vi "HMI.vi"() -> ()   [LabVIEW 2019]
uses:
  Hardware/PfeifferTC110Cmds.ctl
  Hardware/PfeifferMVP15Cmds.ctl
  <vilib>/Utility/miscctls.llb/LVPointTypeDef.ctl
  <vilib>/NI/AMC/Read Termination Message.vi
  <vilib>/NI/AMC/Create Single Message.vi
  <vilib>/NI/AMC/Update Message Routing Info.vi
  <vilib>/NI/AMC/Send Message.vi
  <vilib>/NI/AMC/Globals.vi
  <vilib>/NI/AMC/AMC.lvlib
  <instrlib>/Pfeiffer Vacuum/Pfeiffer Vacuum.lvlib
panel:
  out "status":string
  in  "stop":bool
  in  "Tab Control":enum32{"RGAs", "Gas Flow", "Alarms", "Page 3"}(tab)
  in  "Ring":u16(ring)
  in  "Ack Errors":bool
  out "MainMVP  OpHrs":i32 caption="Op Hrs"
  out "MainMVP  Set Pnt RPM":i32 caption="Set Pnt RPM"
  out "Main Firm MVP":string caption="Firmware"
  out "Main Model MVP":string caption="Model"
  out "Load At Nominal":bool caption="At Nominal"
  out "Main At Nominal":bool caption="At Nominal"
  out "Main Control °C 3":i32(slide) caption="Control °C" scale=0.0..60.0
  out "Main Control °C 2":i32(slide) caption="Control °C" scale=0.0..60.0
  out "Load TMP °C":i32(slide) caption="TMP °C" scale=0.0..60.0
  out "Main TMP °C":i32(slide) caption="TMP °C" scale=0.0..60.0
  out "Load Set Pnt RPM":i32 caption="Set Pnt RPM"
  out "Main Set Pnt RPM":i32 caption="Set Pnt RPM"
  out "Load Cycles":i32 caption="Cycles"
  out "Main Cycles":i32 caption="Cycles"
  out "Load Model":string caption="Model"
  out "Main Model":string caption="Model"
  out "LoadErrorCode 2":string caption="Current Error Code"
  out "MainErrorCode":string caption="Current Error Code"
  out "Load Watts":dbl(knob) caption="Watts" scale=0.0..100.0
  out "Main Watts":dbl(knob) caption="Watts" scale=0.0..100.0
  out "Load RPM":dbl(knob) caption="RPM" scale=0.0..100000.0
  out "Main RPM":dbl(knob) caption="RPM" scale=0.0..100000.0
  in  "Load TMP Standby":bool caption="TMP Standby"
  in  "Main TMP Standby":bool caption="TMP Standby"
  in  "Load TMP Run":bool caption="TMP Run"
  in  "Main TMP Run":bool caption="TMP Run"
  out "MVP RPM":i32(knob) caption="RPM" scale=0.0..2500.0
  out "MVP Watts":i32(knob) caption="Watts" scale=0.0..100.0
  out "Load TMP °C 2":i32(slide) caption="Pmp °C" scale=0.0..60.0
  out "MVPErrorCode":string caption="Current Error Code"
  in  "Main MVP Run":bool caption="MVP Run"
  in  "MainMVP Standby":bool caption="MVP Standby"
  out "P LL":dbl format="%#_2e"
  out "Boolean 6":bool
  out "Boolean 5":bool
  out "Boolean 2":bool
  out "Watts 5":i16 caption="Volts"
  out "RF Fwd":i16
  out "RF Rlfctd":i16
  out "RF Vdc":i16
  out "Watts 4":i16 caption="Watts"
  out "Boolean 32":bool
  out "Boolean 31":bool
  out "Boolean 30":bool
  out "Boolean 29":bool
  out "Boolean 15":bool
  out "Boolean 14":bool
  out "Boolean 13":bool
  out "Boolean 12":bool
  out "Boolean 11":bool
  out "Boolean 10":bool
  out "Boolean 8":bool
  out "Watts":dbl
  out "Watts":dbl
  out "Watts":dbl
  in  "GV4":bool
  in  "GV3":bool
  in  "GV2":bool
  in  "GV1":bool
  out "Boolean":bool
  out "Unload Ch Pressure in Torr":dbl format="%.2e"
  out "MFV1 Chamber Access":bool
  out "Boolean 9":bool
  out "Boolean 7":bool
  out "Ar to MFV1":bool
  out "O2 to MFV1":bool
  out "Boolean 3":bool
  out "MFC2 Gas Spply":bool
  out "IG MFCs to GD":bool
  out "MFC3 Gas Spply":bool
  in  "GD On":bool
  in  "Blank Button 2":bool
  out "IG Chamber Access":bool
  out "MFC1":i16
  out "MFC2":sgl format="%.1f"
  out "MFC3":sgl format="%.1f"
  out "MFC3 Total":sgl format="%.1f"
  out "MFC2 Total":sgl format="%.1f"
  out "Boolean 4":bool
  in  "Blank Button 3":bool
  out "To RGA":bool
  out "Boolean 16":bool
  out "Ar Supply Target 1":bool
  out "MFC4":sgl format="%.1f"
  out "Boolean 17":bool
  out "Targ 1 Total":sgl format="%.1f"
  in  "Blank Button 4":bool
  out "Ar Supply Target 2":bool
  out "MFC5":sgl format="%.1f"
  out "Boolean 18":bool
  out "Targ 2 Total":sgl format="%.1f"
  in  "Blank Button 5":bool
  out "Ar Supply Target 3":bool
  out "MFC6":sgl format="%.1f"
  out "Boolean 19":bool
  out "Targ 3 Total":sgl format="%.1f"
  out "To RGA Main":bool caption="To RGA"
  out "N2 Vent":bool
  out "Atm Vent":bool
  out "Boolean 20":bool
  out "Boolean 21":bool
  out "Boolean 22":bool
  out "Turbo MV1":bool
  in  "LD MV1":bool
  out "Throttle Pos":dbl(knob) scale=0.0..100.0
  out "N2 Vent 2":bool caption="N2 Vent"
  out "Atm Vent 2":bool caption="Atm Vent"
  out "Boolean 23":bool
  out "Boolean 24":bool
  out "Boolean 25":bool
  out "N2 Vent 3":bool caption="N2 Vent"
  out "Atm Vent 3":bool caption="Atm Vent"
  out "Boolean 26":bool
  out "Boolean 27":bool
  out "Boolean 28":bool
  out "PLC":bool
  out "RV1":bool
  out "RV1 2":bool caption="RV3"
  out "P Mn":dbl format="%.2e"
  out "UL_vent_TO":bool
  out "UL_Rough_TO":bool
  out "RV3_Incorr_Op/CL":bool
  out "RV1_Incorr_Op/CL":bool
  out "RF_disch_MV1_Cl":bool
  out "MV1_Incorr_Op/CL":bool
  out "LL_vent_TO":bool
  out "LL_Rough_TO":bool
  out "LL_pumpdn_TO":bool
  out "FV2_Incorr_Op/CL":bool
  out "FV1_Incorr_Op/CL":bool
  out "Chmbr_vent_TO":bool
  out "Chmbr_Rough_TO":bool
  out "TMP2":bool
  out "TMP1":bool
  out "DP2":bool
  out "DP1":bool
  out "DC2B L/H Lim":bool
  out "DC2A L/H Lim":bool
  out "DC1B L/H Lim":bool
  out "DC1A L/H Lim":bool
  out "RF VDC":bool
  out "RF REV Lim":bool
  out "RF FWD Lim":bool
  out "DP3":bool
  out "RF":bool
  # "Main Chamber RGA"
  # "Load Lock RGA"
  # "Main RGA MVP"
  # "Std L"
  # "Std L"
  # "Std L"
  # "Open"
  # "Closed"
  # "SCCM"
  # "SCCM"
  # "SCCM"
  # "SCCM"
  # "Main Ch Pressure \n in Torr"
  # "Std L"
  # "SCCM"
  # "Std L"
  # "SCCM"
  # "Vacuum Alarms"
  # "Sput/Gauge Alarms"
  # "Transport Alarms"
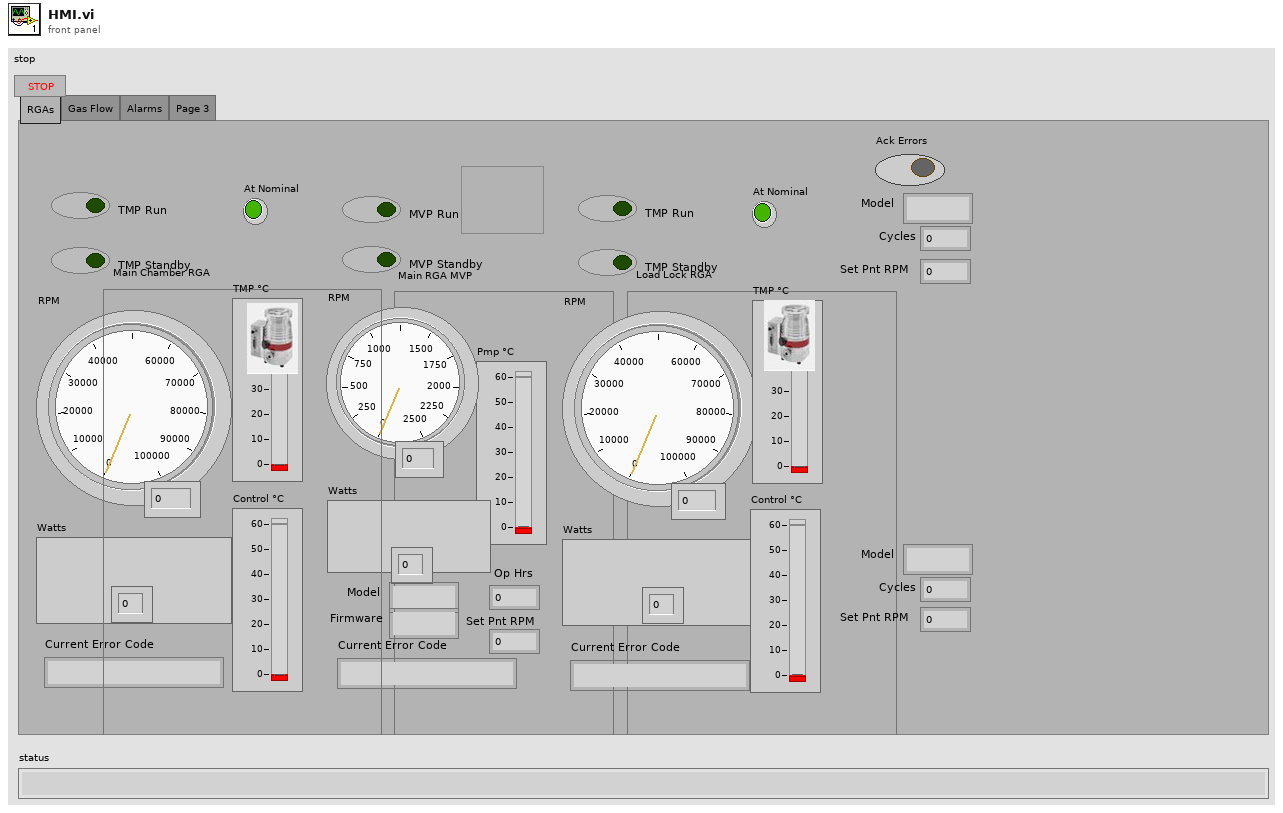
[diagram p1: front panel]
types:
  T1 = typedef "AMC.lvlib/Message Queue.ctl" = refnum<queue>
  T2 = typedef "PfeifferTC110Cmds.ctl" = enum16{"Standby", "AckError", "Run", "Motor", "SpdSwPtAtt", "ErrorCode", "OvTempElec", "OvTempPump", "SetSpdAtt", "PumpAccel", "ActualSpdHz", "DrvCurrent", "OpHrsPump", "FwVersion", "DrvVoltage", "OpHrsElec", "NominalSpd", "DrvPower", "PumpCycles", "TempElec", "TempPmpBot", "AccelDecel", "TempBearing", "TempMotor", "ElecName", "HWVersion", "SetRotSpdRPM", "ActualSpdRPM", "NominalSpdRPM"}
  T3 = typedef "PfeifferMVP15Cmds.ctl" = enum16{"Standby", "Run", "AckError", "ErrorCode", "ActualSpdHz", "DrvCurrent", "OpHrsPump", "FwVersion", "DrvVoltage", "NominalSpdHz", "DrvPower", "ElecName", "HWVersion", "ActualSpdRPM", "NominalSpdRPM", "TempPump"}
  T4 = typedef "LVPointTypeDef.ctl" = cluster{"Horizontal":i16, "Vertical":i16}
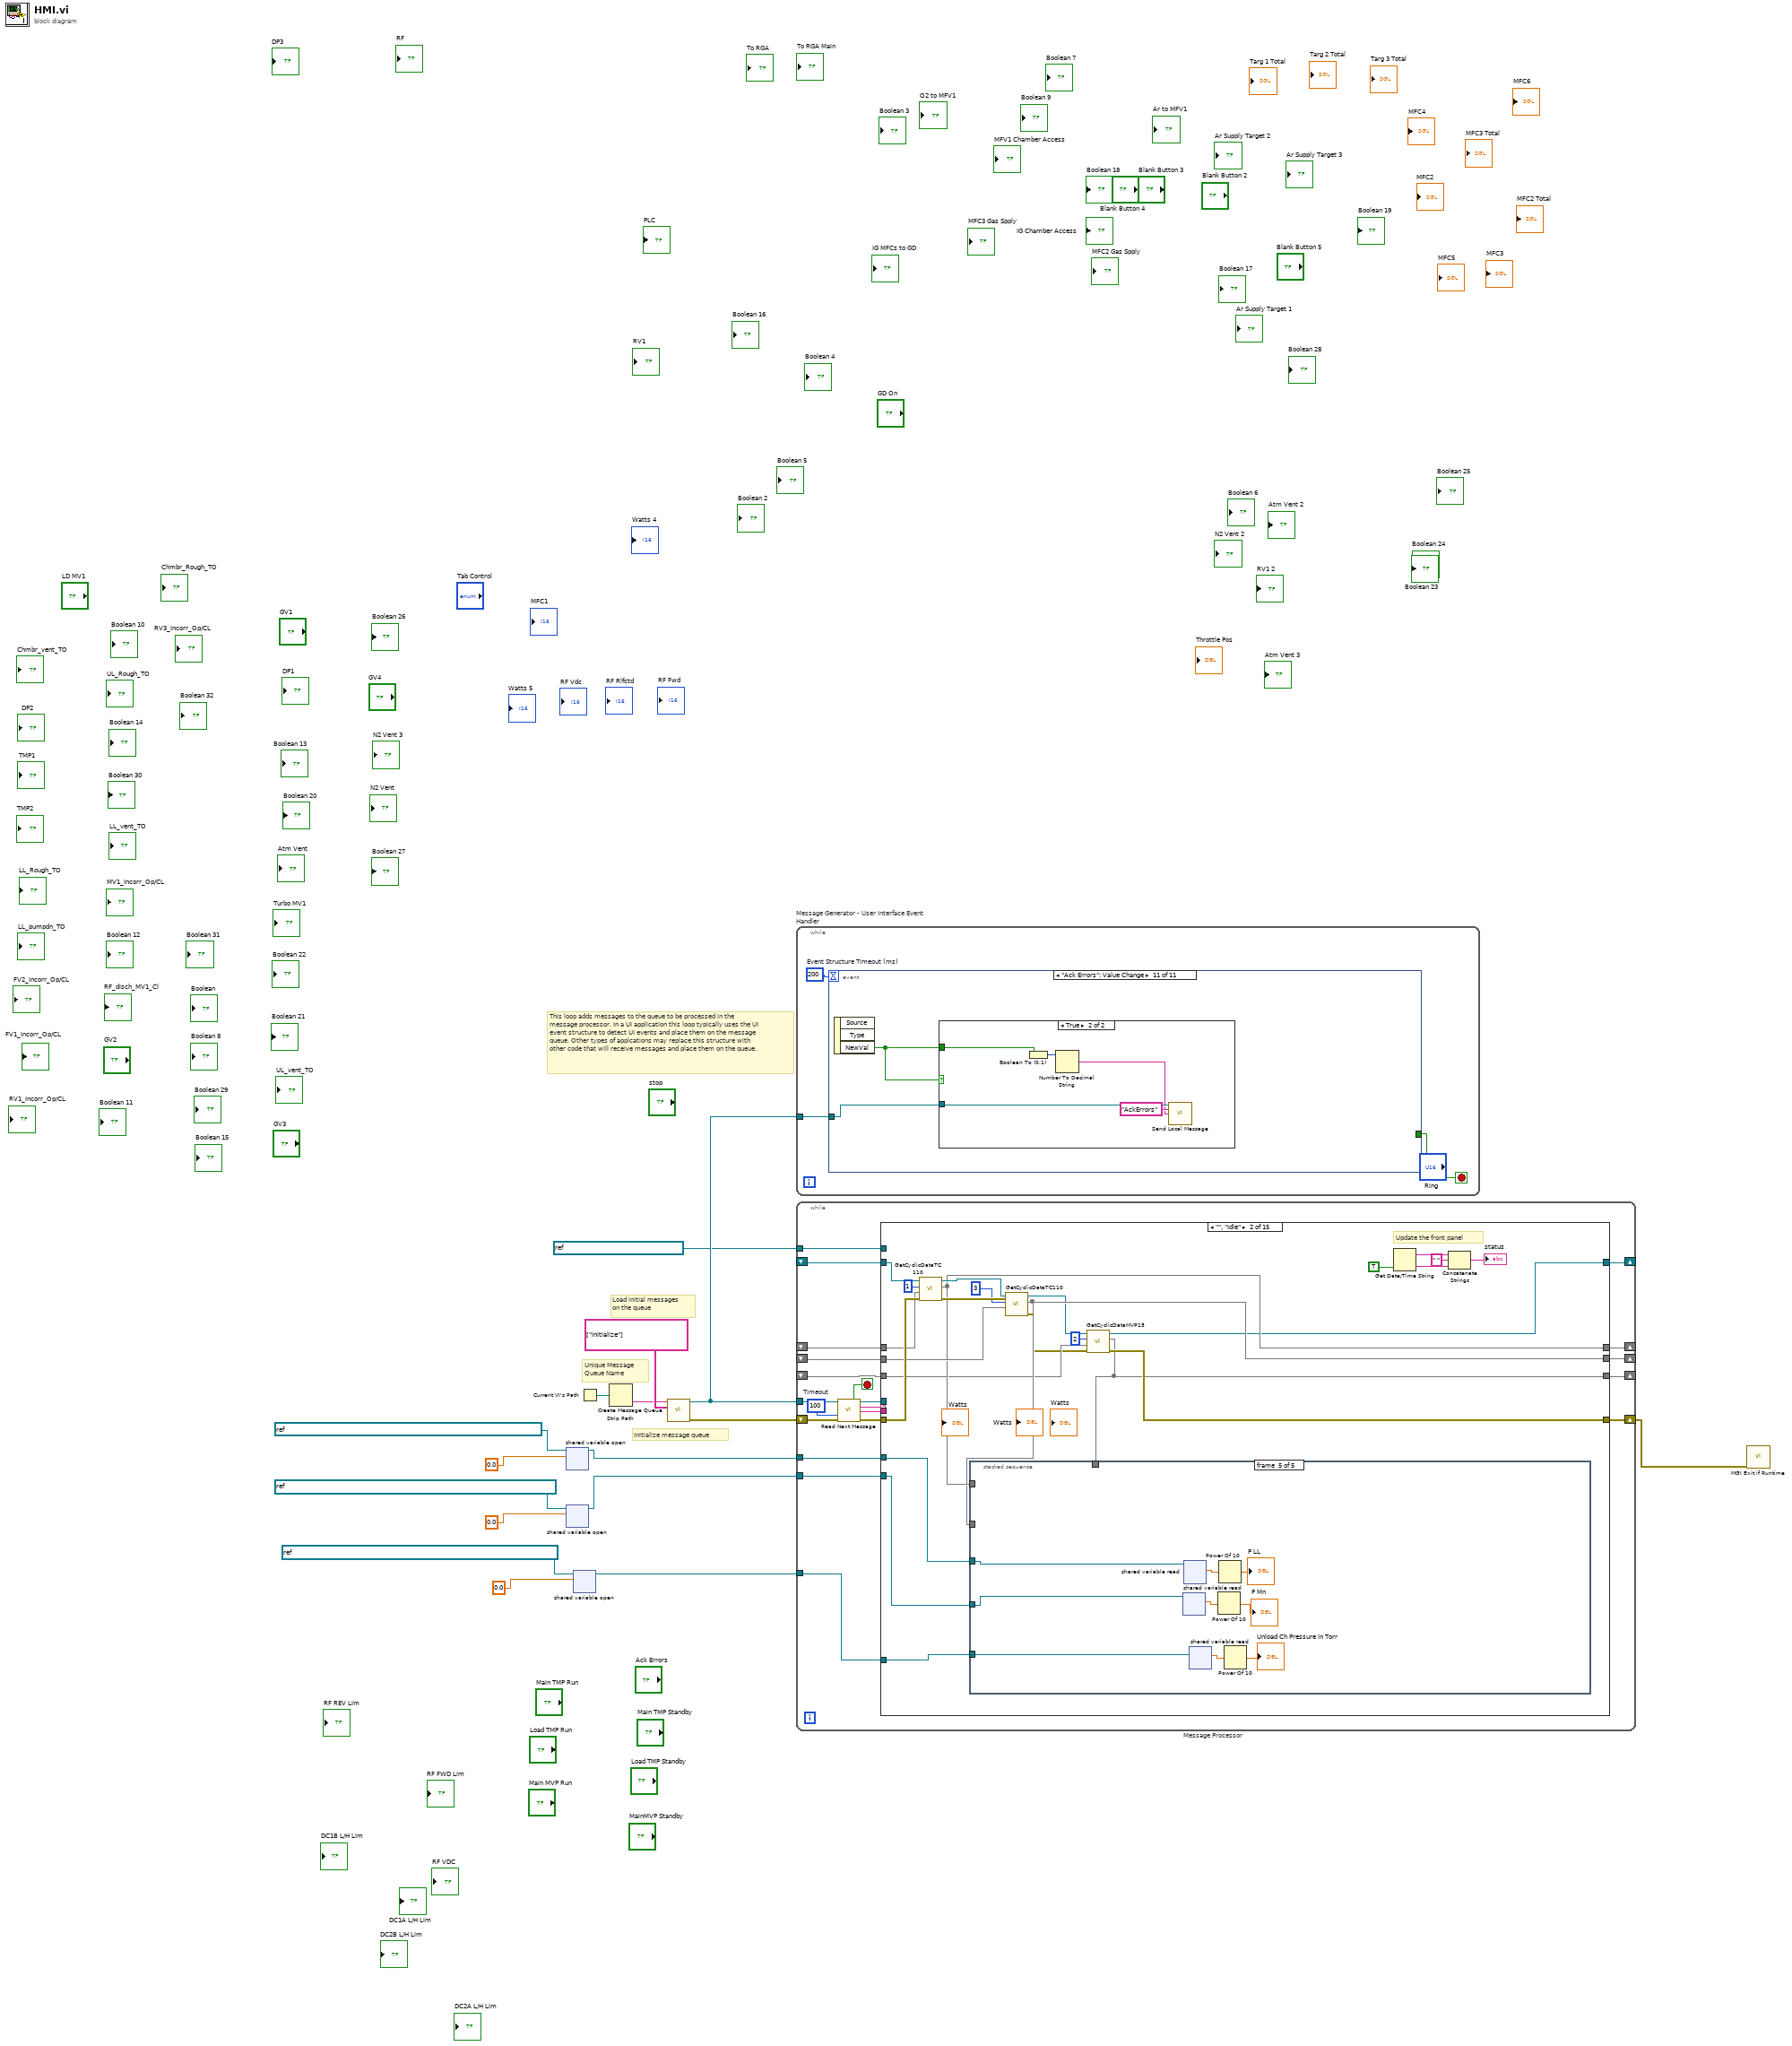
[diagram p0: block diagram]
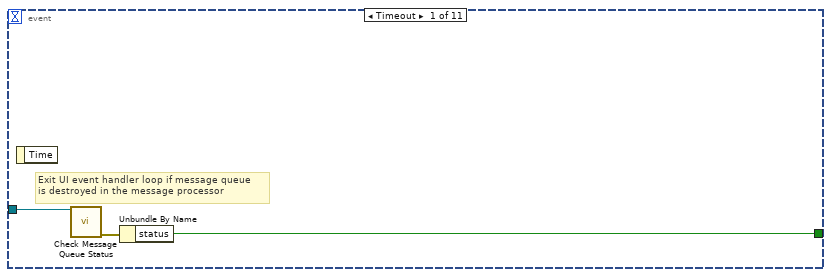
[diagram p2: hidden frame]
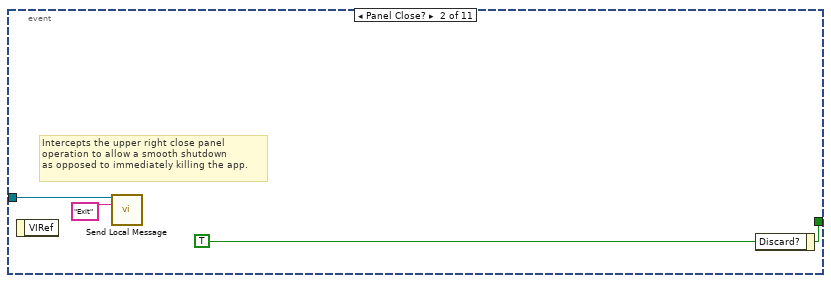
[diagram p3: hidden frame]
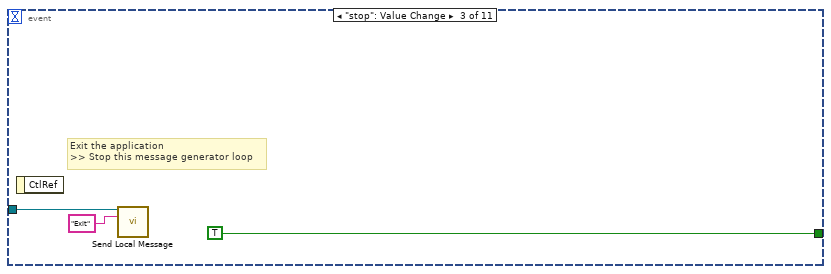
[diagram p4: hidden frame]
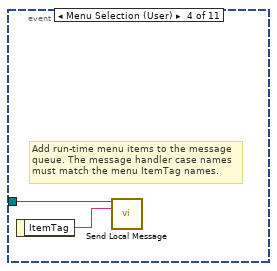
[diagram p5: hidden frame]
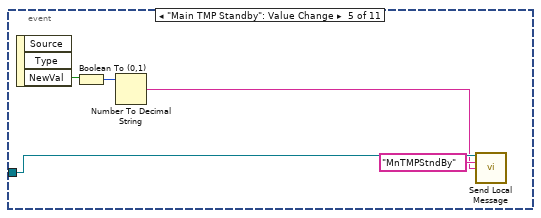
[diagram p6: hidden frame]
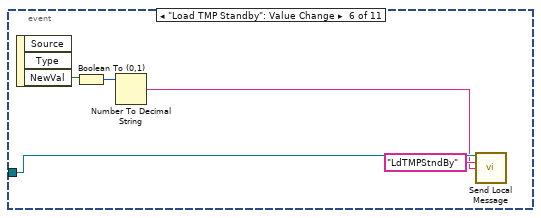
[diagram p7: hidden frame]
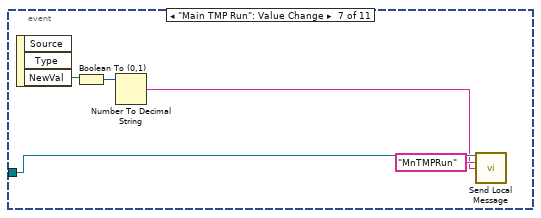
[diagram p8: hidden frame]
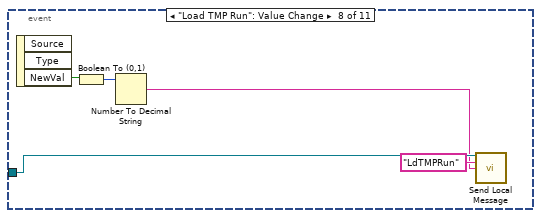
[diagram p9: hidden frame]
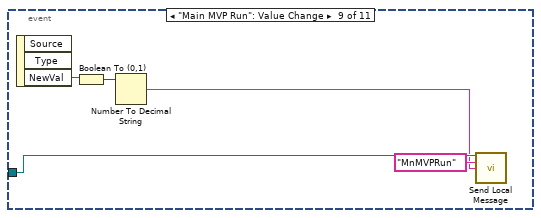
[diagram p10: hidden frame]
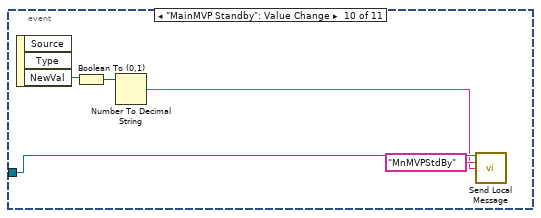
[diagram p11: hidden frame]
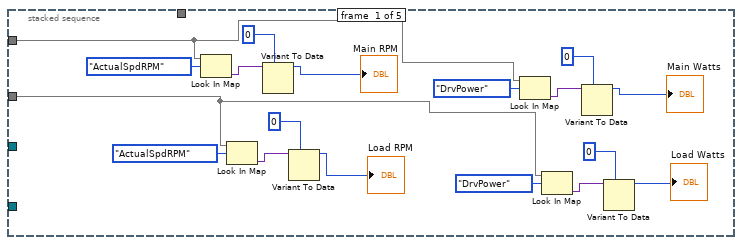
[diagram p14: hidden frame]
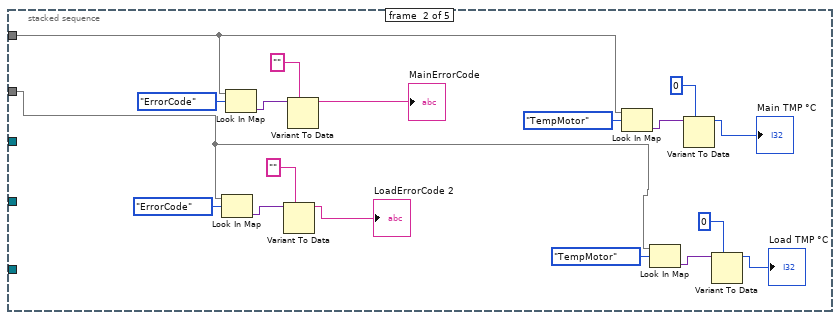
[diagram p15: hidden frame]
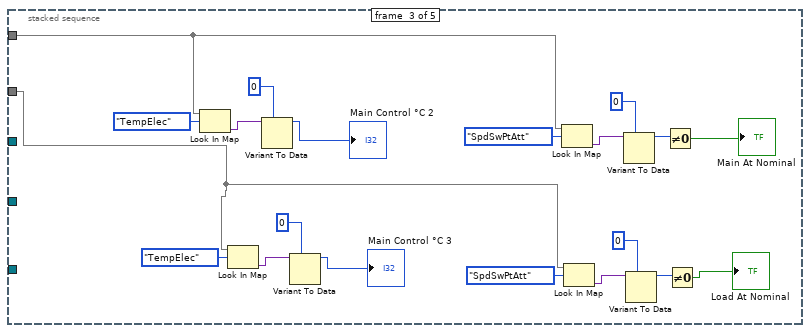
[diagram p16: hidden frame]
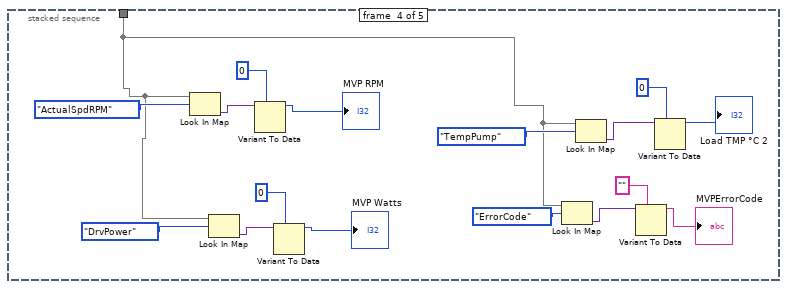
[diagram p17: hidden frame]
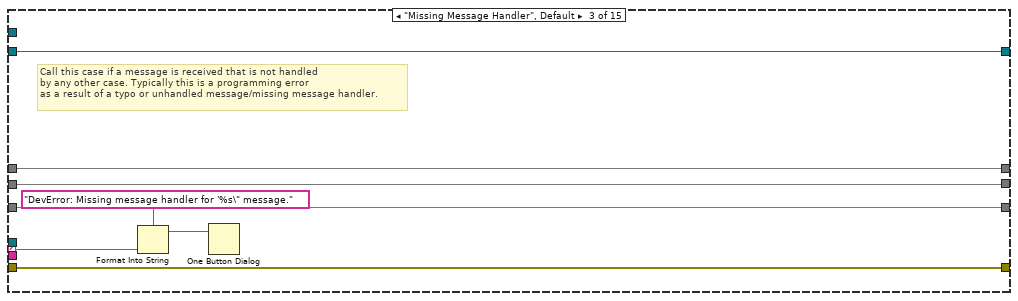
[diagram p18: hidden frame]
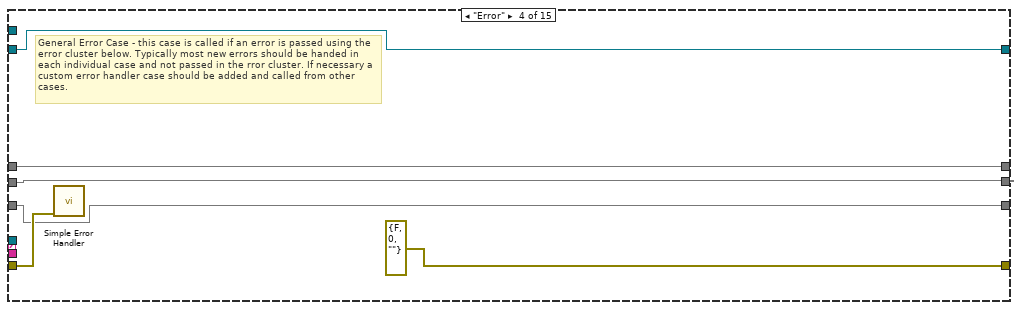
[diagram p19: hidden frame]
diagram:
  # "This loop adds messages to the queue to be processed in the message processor. In a UI application this loop typically uses the UI event structure to detect UI events and place them on the message queue. Other types of applcations may replace this structure with other code that will receive messages and place them on the queue."
  # "Initialize message queue"
  # "Unique Message\nQueue Name"
  # "Load initial messages\non the queue"
  n1 = shared-variable-open(refnum<k21> "ni.var.psp://huniopc01/CDL0097 scada tags/Load_Lock_Pressure" ("shared variable refnum in"), 0.0) -> (w5:refnum<k21>)  [unwired: 2 in, 1 out]
  n2 = shared-variable-open(refnum<k21> "ni.var.psp://huniopc01/CDL0097 scada tags/Main_Chamber_Log10P" ("shared variable refnum in"), 0.0) -> (w4:refnum<k21>)  [unwired: 2 in, 1 out]
  n3 = shared-variable-open(refnum<k21> "ni.var.psp://huniopc01/CDL0097 scada tags/Unload_Lock_Pressure" ("shared variable refnum in"), 0.0) -> (w1:refnum<k21>)  [unwired: 2 in, 1 out]
  n4 = Current VI's Path() -> (path=w12:path)
  n5 = Strip Path(path=w12) -> (name=w15:string)  [unwired: 1 out]
  n6 = call <vilib>:"Create Message Queue.vi"("message queue name"=w15, "initial message names"=string[] ["Initialize"]) -> ("message queue out"=w14:T1, "error out"=w13:errorcluster)  [unwired: 12 in]
  n7 = while "Message Generator - User Interface Event Handler" {
    tunnel: w14 -> [w17]
    stop <- w18 stop-if-true
    w19 = 200  # Event Structure Timeout (ms)
    n8 = event shown="[10] \"Ack Errors\": Value Change" {
      selector: _ -> [_ _ _ _ _ _ _ _ _ _ _]
      dyn-events: _ -> [_ _ _ _ _ _ _ _ _ _ _]
      timeout: w19 -> [_ _ _ _ _ _ _ _ _ _ _]
      tunnel: [w20 w25 TRUE ("Discard?") _ _ _ _ _ _ _ _] -> w18
      tunnel: w17 -> [w21 w23 w26 w29 w35 w40 w45 w50 w55 w60 w62]
      event Timeout {
        # "Exit UI event handler loop if message queue\nis destroyed in the message processor"
        n9 = event-data() -> ()  [unwired: 2 out]
        n10 = call <vilib>:"Check Message Queue Status.vi"("message queue in"=w21) -> ("error out"=w22:errorcluster)  [unwired: 10 in, 4 out]
        n11 = Unbundle By Name(w22) -> ("status"=w20:bool)
      }
      event Panel Close? {
        w25 = TRUE ("Discard?")
        # "Intercepts the upper right close panel\noperation to allow a smooth shutdown\nas opposed to immediately killing the app."
        n12 = event-data() -> ()  [unwired: 2 out]
        n13 = call <vilib>:"Send Local Message.vi"("message queue in"=w23, "message name"="Exit") -> ()  [unwired: 11 in, 3 out]
        n14 = event-data("Discard?"=w25) -> ()  [unwired: 1 in, 1 out]
      }
      event "stop": Value Change {
        # "Exit the application\n>> Stop this message generator loop"
        n15 = event-data() -> ()  [unwired: 2 out]
        n16 = call <vilib>:"Send Local Message.vi"("message queue in"=w26, "message name"="Exit") -> ()  [unwired: 11 in, 3 out]
      }
      event Menu Selection (User) {
        # "Add run-time menu items to the message\nqueue. The message handler case names must match the menu ItemTag names."
        n17 = event-data() -> ("ItemTag"=w30:string)  [unwired: 1 out]
        n18 = call <vilib>:"Send Local Message.vi"("message queue in"=w29, "message name"=w30) -> ()  [unwired: 11 in, 3 out]
      }
      event "Main TMP Standby": Value Change {
        n19 = event-data() -> ("NewVal"=w34:bool)  [unwired: 3 out]
        n20 = Boolean To (0,1)(Boolean=w34) -> (0, 1=w32:i16)
        n21 = Number To Decimal String(number=w32) -> (decimal integer string=w31:string)  [unwired: 1 in]
        n22 = call <vilib>:"Send Local Message.vi"("message queue in"=w35, "message name"="MnTMPStndBy", "message value"=w31) -> ()  [unwired: 10 in, 3 out]
      }
      event "Load TMP Standby": Value Change {
        n23 = event-data() -> ("NewVal"=w39:bool)  [unwired: 3 out]
        n24 = Boolean To (0,1)(Boolean=w39) -> (0, 1=w37:i16)
        n25 = Number To Decimal String(number=w37) -> (decimal integer string=w36:string)  [unwired: 1 in]
        n26 = call <vilib>:"Send Local Message.vi"("message queue in"=w40, "message name"="LdTMPStndBy", "message value"=w36) -> ()  [unwired: 10 in, 3 out]
      }
      event "Main TMP Run": Value Change {
        n27 = event-data() -> ("NewVal"=w44:bool)  [unwired: 3 out]
        n28 = Boolean To (0,1)(Boolean=w44) -> (0, 1=w42:i16)
        n29 = Number To Decimal String(number=w42) -> (decimal integer string=w41:string)  [unwired: 1 in]
        n30 = call <vilib>:"Send Local Message.vi"("message queue in"=w45, "message name"="MnTMPRun", "message value"=w41) -> ()  [unwired: 10 in, 3 out]
      }
      event "Load TMP Run": Value Change {
        n31 = event-data() -> ("NewVal"=w49:bool)  [unwired: 3 out]
        n32 = Boolean To (0,1)(Boolean=w49) -> (0, 1=w47:i16)
        n33 = Number To Decimal String(number=w47) -> (decimal integer string=w46:string)  [unwired: 1 in]
        n34 = call <vilib>:"Send Local Message.vi"("message queue in"=w50, "message name"="LdTMPRun", "message value"=w46) -> ()  [unwired: 10 in, 3 out]
      }
      event "Main MVP Run": Value Change {
        n35 = event-data() -> ("NewVal"=w54:bool)  [unwired: 3 out]
        n36 = Boolean To (0,1)(Boolean=w54) -> (0, 1=w52:i16)
        n37 = Number To Decimal String(number=w52) -> (decimal integer string=w51:string)  [unwired: 1 in]
        n38 = call <vilib>:"Send Local Message.vi"("message queue in"=w55, "message name"="MnMVPRun", "message value"=w51) -> ()  [unwired: 10 in, 3 out]
      }
      event "MainMVP Standby": Value Change {
        n39 = event-data() -> ("NewVal"=w59:bool)  [unwired: 3 out]
        n40 = Boolean To (0,1)(Boolean=w59) -> (0, 1=w57:i16)
        n41 = Number To Decimal String(number=w57) -> (decimal integer string=w56:string)  [unwired: 1 in]
        n42 = call <vilib>:"Send Local Message.vi"("message queue in"=w60, "message name"="MnMVPStdBy", "message value"=w56) -> ()  [unwired: 10 in, 3 out]
      }
      event "Ack Errors": Value Change {
        n43 = event-data() -> ("NewVal"=w61:bool)  [unwired: 3 out]
        n44 = case shown="True" w61 {
          tunnel: w62 -> [_ w67]
          tunnel: w61 -> [_ w66]
          frame False {
          }
          frame True {
            n45 = Boolean To (0,1)(Boolean=w66) -> (0, 1=w64:i16)
            n46 = Number To Decimal String(number=w64) -> (decimal integer string=w63:string)  [unwired: 1 in]
            n47 = call <vilib>:"Send Local Message.vi"("message queue in"=w67, "message name"="AckErrors", "message value"=w63) -> ()  [unwired: 10 in, 3 out]
          }
        }
      }
    }
  }
  n48 = while "Message Processor" {
    shift-left: w13 -> [w84]
    shift-right: [w88] -> w10
    tunnel: w14 -> [w85]
    tunnel: refnum<visa-resource-name> "visa://Z016807/ASRL5::INSTR" ("VISA resource name") -> [w79]
    shift-right: [w78] -> _
    shift-left: _ -> [w75]
    shift-right: [w77] -> _
    shift-left: _ -> [w73]
    shift-right: [w76] -> _
    shift-left: _ -> [w74]
    tunnel: w5 -> [w72]
    tunnel: w4 -> [w71]
    shift-right: [w70] -> _
    shift-left: _ -> [w69]
    tunnel: w1 -> [w68]
    stop <- w87 stop-if-true
    w80 = 100  # Timeout
    n49 = call <vilib>:"Read Next Message.vi"("message queue in"=w85, "timeout (1 ms)"=w80, "error in"=w84) -> ("exit process?"=w87:bool, "message queue out"=w86:T1, "message name"=w82:string, "message value"=w81:string, "error out"=w83:errorcluster)  [unwired: 5 in, 3 out]
    n50 = case shown="\"\", \"Idle\"" w82 {
      selector: w82 -> [_ _ w207 _ _ _ _ _ _ _ _ _ _ _ _]
      tunnel: w86 -> [_ _ _ _ _ _ w333 _ _ _ _ _ _ _ _]
      tunnel: w83 -> [w93 w111 w208 w213 w219 w245 w334 w340 w351 w366 w381 w396 w406 w421 w444]
      tunnel: [w93 w96 w208 errorcluster {"status"=FALSE, "code"=0, "source"=""} ("error out") w219 w222 w331 w340 w343 w358 w373 w388 w401 w416 w435] -> w88
      tunnel: w81 -> [_ _ _ _ _ _ _ _ w349 w364 w379 w394 w414 w429 _]
      tunnel: w79 -> [_ _ _ _ _ w246 _ _ _ _ _ _ _ _ _]
      tunnel: [w92 w100 w204 w210 w216 w221 w330 w337 w350 w365 w380 w395 w410 w425 w433] -> w78
      tunnel: [w90 w104 w202 w211 w218 w230 w328 w339 w355 w370 w385 w400 w415 w430 w442] -> w77
      tunnel: [w91 w105 w203 w212 w217 w231 w329 w338 w342 w357 w372 w387 w412 w427 w443] -> w76
      tunnel: w75 -> [w92 w113 w204 w210 w216 _ w330 w337 w353 w368 w383 w398 w411 w426 w446]
      tunnel: w74 -> [w91 w110 w203 w212 w217 w233 w329 w338 w346 w361 w376 w391 w412 w427 w443]
      tunnel: w73 -> [w90 w108 w202 w211 w218 w232 w328 w339 w355 w370 w385 w400 w415 w430 w442]
      tunnel: w72 -> [_ w102 _ _ _ _ _ _ _ _ _ _ _ _ _]
      tunnel: w71 -> [_ w103 _ _ _ _ _ _ _ _ _ _ _ _ _]
      tunnel: [w89 w95 w201 w209 w215 w220 w327 w336 w341 w356 w371 w386 w402 w417 w434] -> w70
      tunnel: w69 -> [w89 w99 w201 w209 w215 _ w327 w336 w341 w356 w371 w386 w404 w419 w434]
      tunnel: w68 -> [_ w94 _ _ _ _ _ _ _ _ _ _ _ _ _]
      frame "---------- Framework Operations ----------" {
        # "Dummy case to add a seperator in the Case Structure menu"
      }
      frame "", "Idle" {
        # "Update the front panel"
        n51 = call "GetCyclicDataTC110.vi"("error in (no error)"=w111, "Map"=w110, "Adress of unit"=u16 1, "VISA Refnum in"=w113) -> ("error out"=w109:errorcluster, "Map 2"=w105:map{T2, variant}, "VISA session out"=w106:refnum<visa-resource-name>)  [unwired: 5 in]
        n52 = call "GetCyclicDataTC110.vi"("error in (no error)"=w109, "Map"=w108, "Adress of unit"=u16 3, "VISA Refnum in"=w106) -> ("error out"=w97:errorcluster, "Map 2"=w104:map{T2, variant}, "VISA session out"=w101:refnum<visa-resource-name>)  [unwired: 5 in]
        n53 = call "GetCyclicDataMVP15.vi"("error In"=w97, "Map In"=w99, "Adress"=u16 2, "VISA session"=w101) -> ("error out"=w96:errorcluster, "Map"=w95:map{T3, variant}, "VISA session Out"=w100:refnum<visa-resource-name>)  [unwired: 5 in]
        n54 = stacked-sequence {
          tunnel: w105 -> [w125 w140 w164 _ _]
          tunnel: w104 -> [w120 w139 w156 _ _]
          tunnel: w103 -> [_ _ _ _ w195]
          tunnel: w102 -> [_ _ _ _ w196]
          tunnel: w95 -> [_ _ _ w178 _]
          tunnel: w94 -> [_ _ _ _ w193]
          frame #0 {
            n55 = Look In Map(map=w125, key=PfeifferTC110Cmds."ActualSpdRPM") -> (value=w134:variant)  [unwired: 1 in, 1 out]
            n56 = Look In Map(map=w120, key=PfeifferTC110Cmds."ActualSpdRPM") -> (value=w130:variant)  [unwired: 1 in, 1 out]
            n57 = Variant To Data(type=0, Variant=w134) -> (data=→"Main RPM":i32)  [unwired: 1 in, 1 out]
            n58 = Variant To Data(type=0, Variant=w130) -> (data=→"Load RPM":i32)  [unwired: 1 in, 1 out]
            n59 = Look In Map(map=w125, key=PfeifferTC110Cmds."DrvPower") -> (value=w126:variant)  [unwired: 1 in, 1 out]
            n60 = Look In Map(map=w120, key=PfeifferTC110Cmds."DrvPower") -> (value=w121:variant)  [unwired: 1 in, 1 out]
            n61 = Variant To Data(type=0, Variant=w126) -> (data=→"Main Watts":i32)  [unwired: 1 in, 1 out]
            n62 = Variant To Data(type=0, Variant=w121) -> (data=→"Load Watts":i32)  [unwired: 1 in, 1 out]
          }
          frame #1 {
            n63 = Look In Map(map=w139, key=PfeifferTC110Cmds."ErrorCode") -> (value=w149:variant)  [unwired: 1 in, 1 out]
            n64 = Look In Map(map=w140, key=PfeifferTC110Cmds."ErrorCode") -> (value=w153:variant)  [unwired: 1 in, 1 out]
            n65 = Variant To Data(type="", Variant=w149) -> (data=→"LoadErrorCode 2":string)  [unwired: 1 in, 1 out]
            n66 = Variant To Data(type="", Variant=w153) -> (data=→"MainErrorCode":string)  [unwired: 1 in, 1 out]
            n67 = Look In Map(map=w140, key=PfeifferTC110Cmds."TempMotor") -> (value=w145:variant)  [unwired: 1 in, 1 out]
            n68 = Look In Map(map=w139, key=PfeifferTC110Cmds."TempMotor") -> (value=w142:variant)  [unwired: 1 in, 1 out]
            n69 = Variant To Data(type=0, Variant=w145) -> (data=→"Main TMP °C":i32)  [unwired: 1 in, 1 out]
            n70 = Variant To Data(type=0, Variant=w142) -> (data=→"Load TMP °C":i32)  [unwired: 1 in, 1 out]
          }
          frame #2 {
            n71 = Look In Map(map=w164, key=PfeifferTC110Cmds."TempElec") -> (value=w173:variant)  [unwired: 1 in, 1 out]
            n72 = Look In Map(map=w156, key=PfeifferTC110Cmds."TempElec") -> (value=w170:variant)  [unwired: 1 in, 1 out]
            n73 = Variant To Data(type=0, Variant=w173) -> (data=→"Main Control °C 2":i32)  [unwired: 1 in, 1 out]
            n74 = Variant To Data(type=0, Variant=w170) -> (data=→"Main Control °C 3":i32)  [unwired: 1 in, 1 out]
            n75 = Look In Map(map=w164, key=PfeifferTC110Cmds."SpdSwPtAtt") -> (value=w163:variant)  [unwired: 1 in, 1 out]
            n76 = Look In Map(map=w156, key=PfeifferTC110Cmds."SpdSwPtAtt") -> (value=w158:variant)  [unwired: 1 in, 1 out]
            n77 = Variant To Data(type=0, Variant=w163) -> (data=w162:i32)  [unwired: 1 in, 1 out]
            n78 = Variant To Data(type=0, Variant=w158) -> (data=w157:i32)  [unwired: 1 in, 1 out]
            n79 = Not Equal To 0?(x=w162) -> (x != 0?=→"Main At Nominal":bool)
            n80 = Not Equal To 0?(x=w157) -> (x != 0?=→"Load At Nominal":bool)
          }
          frame #3 {
            n81 = Look In Map(map=w178, key=PfeifferMVP15Cmds."ActualSpdRPM") -> (value=w190:variant)  [unwired: 1 in, 1 out]
            n82 = Look In Map(map=w178, key=PfeifferMVP15Cmds."DrvPower") -> (value=w186:variant)  [unwired: 1 in, 1 out]
            n83 = Variant To Data(type=0, Variant=w190) -> (data=→"MVP RPM":i32)  [unwired: 1 in, 1 out]
            n84 = Variant To Data(type=0, Variant=w186) -> (data=→"MVP Watts":i32)  [unwired: 1 in, 1 out]
            n85 = Look In Map(map=w178, key=PfeifferMVP15Cmds."ErrorCode") -> (value=w177:variant)  [unwired: 1 in, 1 out]
            n86 = Look In Map(map=w178, key=PfeifferMVP15Cmds."TempPump") -> (value=w181:variant)  [unwired: 1 in, 1 out]
            n87 = Variant To Data(type="", Variant=w177) -> (data=→"MVPErrorCode":string)  [unwired: 1 in, 1 out]
            n88 = Variant To Data(type=0, Variant=w181) -> (data=→"Load TMP °C 2":i32)  [unwired: 1 in, 1 out]
          }
          frame #4 {
            n89 = shared-variable-read(w195) -> (w198:dbl)  [unwired: 1 in, 3 out]
            n90 = shared-variable-read(w196) -> (w200:dbl)  [unwired: 1 in, 3 out]
            n91 = shared-variable-read(w193) -> (w194:dbl)  [unwired: 1 in, 3 out]
            n92 = Power Of 10(x=w198) -> (10^x=→"P Mn":dbl)
            n93 = Power Of 10(x=w200) -> (10^x=→"P LL":dbl)
            n94 = Power Of 10(x=w194) -> (10^x=→"Unload Ch Pressure in Torr":dbl)
          }
        }
        n95 = Get Date/Time String(want seconds? (F)=TRUE) -> (date string=w118:string, time string=w117:string)  [unwired: 2 out]
        n96 = Concatenate Strings(w118, " " ("string"), w117) -> (→"status":string)
      }
      frame "Missing Message Handler", Default {
        # "Call this case if a message is received that is not handled \nby any other case. Typically this is a programming error\nas a result of a typo or unhandled message/missing message handler."
        n97 = Format Into String(format string="DevError: Missing message handler for '%s\" message." ("message"), w207) -> (resulting string=w205:string)  [unwired: 2 in, 1 out]
        n98 = One Button Dialog(message=w205) -> ()  [unwired: 2 out]
      }
      frame "Error" {
        # "General Error Case - this case is called if an error is passed using the error cluster below. Typically most new errors should be handed in each individual case and not passed in the rror cluster. If necessary a custom error handler case should be added and called from other cases."
        n99 = call <vilib>:"Simple Error Handler.vi"("error in (no error)"=w213) -> ()  [unwired: 1 in, 8 out]
      }
      frame "---------- Generic Operations ----------" {
        # "Dummy case to add a seperator in the Case Structure menu"
      }
      frame "Initialize" {
        w225 = u16 2 ("Adress")
        w236 = u16 3 ("Adress of unit")
        w242 = u16 1 ("Adress of unit")
        # "Initialize the state variables and user interface"
        n100 = property on="Pane" class="Pane"("Origin"=T4 {"Horizontal"=0, "Vertical"=0}) -> ()  [unwired: 2 in, 2 out]
        n101 = VISA Open(VISA resource name=w246) -> (VISA resource name=w248:refnum<visa-resource-name>, error out=w247:errorcluster)  [unwired: 4 in]
        n102 = call <instrlib>:"PV Initialize.vi"("error in (no error)"=w247, "VISA session in"=w248) -> ("VISA session out"=w241:refnum<visa-resource-name>)  [unwired: 8 in, 1 out]
        n103 = call "GetInitialDataTC110.vi"("error in (no error)"=w245, "Map"=w233, "Adress of unit"=w242, "VISA Refnum in"=w241) -> ("error out"=w244:errorcluster, "data map"=w235:map{T2, variant}, "VISA session out"=w240:refnum<visa-resource-name>)  [unwired: 5 in]
        n104 = call "GetInitialDataTC110.vi"("error in (no error)"=w244, "Map"=w232, "Adress of unit"=w236, "VISA Refnum in"=w240) -> ("error out"=w243:errorcluster, "data map"=w234:map{T2, variant}, "VISA session out"=w239:refnum<visa-resource-name>)  [unwired: 5 in]
        n105 = call "GetCyclicDataTC110.vi"("error in (no error)"=w243, "Map"=w235, "Adress of unit"=w242, "VISA Refnum in"=w239) -> ("error out"=w238:errorcluster, "Map 2"=w231:map{T2, variant}, "VISA session out"=w237:refnum<visa-resource-name>)  [unwired: 5 in]
        n106 = call "GetCyclicDataTC110.vi"("error in (no error)"=w238, "Map"=w234, "Adress of unit"=w236, "VISA Refnum in"=w237) -> ("error out"=w227:errorcluster, "Map 2"=w230:map{T2, variant}, "VISA session out"=w228:refnum<visa-resource-name>)  [unwired: 5 in]
        n107 = call "GetInitialDataMVP15.vi"("error In"=w227, "Adress"=w225, "VISA session"=w228) -> ("error out"=w223:errorcluster, "Map"=w224:map{T3, variant}, "VISA session Out"=w226:refnum<visa-resource-name>)  [unwired: 6 in]
        n108 = call "GetCyclicDataMVP15.vi"("error In"=w223, "Map In"=w224, "Adress"=w225, "VISA session"=w226) -> ("error out"=w222:errorcluster, "Map"=w220:map{T3, variant}, "VISA session Out"=w221:refnum<visa-resource-name>)  [unwired: 5 in]
        n109 = stacked-sequence {
          tunnel: w231 -> [w256 w278 w290 _ _]
          tunnel: w230 -> [w250 w272 w289 _ _]
          tunnel: w220 -> [_ _ _ w302 w317]
          frame #0 {
            n110 = Look In Map(map=w250, key=PfeifferTC110Cmds."Run") -> (value=w262:variant)  [unwired: 1 in, 1 out]
            n111 = Look In Map(map=w256, key=PfeifferTC110Cmds."Run") -> (value=w269:variant)  [unwired: 1 in, 1 out]
            n112 = Variant To Data(type=0, Variant=w269) -> (data=w267:i32)  [unwired: 1 in, 1 out]
            n113 = Variant To Data(type=0, Variant=w262) -> (data=w263:i32)  [unwired: 1 in, 1 out]
            n114 = Not Equal To 0?(x=w267) -> (x != 0?=w266:bool)
            n115 = Not Equal To 0?(x=w263) -> (x != 0?=w261:bool)
            n116 = local write "Main TMP Run"(w266) -> ()
            n117 = local write "Load TMP Run"(w261) -> ()
            n118 = Look In Map(map=w250, key=PfeifferTC110Cmds."Standby") -> (value=w253:variant)  [unwired: 1 in, 1 out]
            n119 = Variant To Data(type=0, Variant=w253) -> (data=w251:i32)  [unwired: 1 in, 1 out]
            n120 = Look In Map(map=w256, key=PfeifferTC110Cmds."Standby") -> (value=w259:variant)  [unwired: 1 in, 1 out]
            n121 = Not Equal To 0?(x=w251) -> (x != 0?=w249:bool)
            n122 = Variant To Data(type=0, Variant=w259) -> (data=w257:i32)  [unwired: 1 in, 1 out]
            n123 = local write "Load TMP Standby"(w249) -> ()
            n124 = Not Equal To 0?(x=w257) -> (x != 0?=w255:bool)
            n125 = local write "Main TMP Standby"(w255) -> ()
          }
          frame #1 {
            n126 = Look In Map(map=w278, key=PfeifferTC110Cmds."ElecName") -> (value=w287:variant)  [unwired: 1 in, 1 out]
            n127 = Look In Map(map=w272, key=PfeifferTC110Cmds."ElecName") -> (value=w284:variant)  [unwired: 1 in, 1 out]
            n128 = Variant To Data(type="", Variant=w287) -> (data=→"Main Model":string)  [unwired: 1 in, 1 out]
            n129 = Variant To Data(type="", Variant=w284) -> (data=→"Load Model":string)  [unwired: 1 in, 1 out]
            n130 = Look In Map(map=w278, key=PfeifferTC110Cmds."PumpCycles") -> (value=w279:variant)  [unwired: 1 in, 1 out]
            n131 = Look In Map(map=w272, key=PfeifferTC110Cmds."PumpCycles") -> (value=w274:variant)  [unwired: 1 in, 1 out]
            n132 = Variant To Data(type=0, Variant=w279) -> (data=→"Main Cycles":i32)  [unwired: 1 in, 1 out]
            n133 = Variant To Data(type=0, Variant=w274) -> (data=→"Load Cycles":i32)  [unwired: 1 in, 1 out]
          }
          frame #2 {
            n134 = Look In Map(map=w290, key=PfeifferTC110Cmds."NominalSpdRPM") -> (value=w297:variant)  [unwired: 1 in, 1 out]
            n135 = Look In Map(map=w289, key=PfeifferTC110Cmds."NominalSpdRPM") -> (value=w294:variant)  [unwired: 1 in, 1 out]
            n136 = Variant To Data(type=0, Variant=w297) -> (data=→"Main Set Pnt RPM":i32)  [unwired: 1 in, 1 out]
            n137 = Variant To Data(type=0, Variant=w294) -> (data=→"Load Set Pnt RPM":i32)  [unwired: 1 in, 1 out]
          }
          frame #3 {
            n138 = Look In Map(map=w302, key=PfeifferMVP15Cmds."ElecName") -> (value=w314:variant)  [unwired: 1 in, 1 out]
            n139 = Look In Map(map=w302, key=PfeifferMVP15Cmds."FwVersion") -> (value=w310:variant)  [unwired: 1 in, 1 out]
            n140 = Variant To Data(type="", Variant=w314) -> (data=→"Main Model MVP":string)  [unwired: 1 in, 1 out]
            n141 = Variant To Data(type="", Variant=w310) -> (data=→"Main Firm MVP":string)  [unwired: 1 in, 1 out]
            n142 = Look In Map(map=w302, key=PfeifferMVP15Cmds."NominalSpdRPM") -> (value=w305:variant)  [unwired: 1 in, 1 out]
            n143 = Look In Map(map=w302, key=PfeifferMVP15Cmds."OpHrsPump") -> (value=w300:variant)  [unwired: 1 in, 1 out]
            n144 = Variant To Data(type=0, Variant=w305) -> (data=→"MainMVP  Set Pnt RPM":i32)  [unwired: 1 in, 1 out]
            n145 = Variant To Data(type=0, Variant=w300) -> (data=→"MainMVP  OpHrs":i32)  [unwired: 1 in, 1 out]
          }
          frame #4 {
            n146 = Look In Map(map=w317, key=PfeifferMVP15Cmds."Run") -> (value=w324:variant)  [unwired: 1 in, 1 out]
            n147 = Look In Map(map=w317, key=PfeifferMVP15Cmds."Standby") -> (value=w319:variant)  [unwired: 1 in, 1 out]
            n148 = Variant To Data(type=0, Variant=w324) -> (data=w323:i32)  [unwired: 1 in, 1 out]
            n149 = Variant To Data(type=0, Variant=w319) -> (data=w318:i32)  [unwired: 1 in, 1 out]
            n150 = Not Equal To 0?(x=w323) -> (x != 0?=w322:bool)
            n151 = Not Equal To 0?(x=w318) -> (x != 0?=w316:bool)
            n152 = local write "Main MVP Run"(w322) -> ()
            n153 = local write "MainMVP Standby"(w316) -> ()
          }
        }
      }
      frame "Exit" {
        # "Destroy message queue >> this will halt the UI event handler loop"
        # "Stop the VI\n>> Perform any cleanup tasks in this message case.\n>> Clear display before closing."
        n154 = call <vilib>:"Destroy Message Queue.vi"("message queue in"=w333, "error in"=w334) -> ("error out"=w332:errorcluster)  [unwired: 11 in, 2 out]
        n155 = local write "status"("" ("Status")) -> ()
        n156 = call <instrlib>:"PV Close.vi"("VISA session"=w330, "error in (no error)"=w332) -> ("error out"=w331:errorcluster)  [unwired: 13 in]
      }
      frame "---------- Application Operations ----------" {
        # "Dummy case to add a seperator in the Case Structure menu"
      }
      frame "MnTMPStndBy" {
        w345 = PfeifferTC110Cmds."Standby" ("CMD ID")
        # "Add actions to perform in response to Process button being pressed"
        n157 = Decimal String To Number(string=w349) -> (number=w348:i32)  [unwired: 2 in, 1 out]
        n158 = Not Equal To 0?(x=w348) -> (x != 0?=w347:bool)
        n159 = call "PfeifferTC110.vi"("On/off"=w347, "Write?"=TRUE, "error in"=w351, "Adress"=u16 1, "VISA session"=w353, "CMD ID"=w345) -> ("error out"=w343:errorcluster, "Response"=w344:variant, "VISA session out"=w350:refnum<visa-resource-name>)  [unwired: 3 in]
        n160 = Insert Into Map(map in=w346, key=w345, value=w344) -> (map out=w342:map{T2, variant})  [unwired: 2 out]
      }
      frame "MnTMPRun" {
        w360 = PfeifferTC110Cmds."Run" ("CMD ID")
        # "Add actions to perform in response to Process button being pressed"
        n161 = Decimal String To Number(string=w364) -> (number=w363:i32)  [unwired: 2 in, 1 out]
        n162 = Not Equal To 0?(x=w363) -> (x != 0?=w362:bool)
        n163 = call "PfeifferTC110.vi"("On/off"=w362, "Write?"=TRUE, "error in"=w366, "Adress"=u16 1, "VISA session"=w368, "CMD ID"=w360) -> ("error out"=w358:errorcluster, "Response"=w359:variant, "VISA session out"=w365:refnum<visa-resource-name>)  [unwired: 3 in]
        n164 = Insert Into Map(map in=w361, key=w360, value=w359) -> (map out=w357:map{T2, variant})  [unwired: 2 out]
      }
      frame "LdTMPStndBy" {
        w375 = PfeifferTC110Cmds."Standby" ("CMD ID")
        # "Add actions to perform in response to Process button being pressed"
        n165 = Decimal String To Number(string=w379) -> (number=w378:i32)  [unwired: 2 in, 1 out]
        n166 = Not Equal To 0?(x=w378) -> (x != 0?=w377:bool)
        n167 = call "PfeifferTC110.vi"("On/off"=w377, "Write?"=TRUE, "error in"=w381, "Adress"=u16 3, "VISA session"=w383, "CMD ID"=w375) -> ("error out"=w373:errorcluster, "Response"=w374:variant, "VISA session out"=w380:refnum<visa-resource-name>)  [unwired: 3 in]
        n168 = Insert Into Map(map in=w376, key=w375, value=w374) -> (map out=w372:map{T2, variant})  [unwired: 2 out]
      }
      frame "LdTMPRun" {
        w390 = PfeifferTC110Cmds."Run" ("CMD ID")
        # "Add actions to perform in response to Process button being pressed"
        n169 = Decimal String To Number(string=w394) -> (number=w393:i32)  [unwired: 2 in, 1 out]
        n170 = Not Equal To 0?(x=w393) -> (x != 0?=w392:bool)
        n171 = call "PfeifferTC110.vi"("On/off"=w392, "Write?"=TRUE, "error in"=w396, "Adress"=u16 3, "VISA session"=w398, "CMD ID"=w390) -> ("error out"=w388:errorcluster, "Response"=w389:variant, "VISA session out"=w395:refnum<visa-resource-name>)  [unwired: 3 in]
        n172 = Insert Into Map(map in=w391, key=w390, value=w389) -> (map out=w387:map{T2, variant})  [unwired: 2 out]
      }
      frame "MnMVPRun" {
        w403 = PfeifferMVP15Cmds."Run" ("Cmd")
        # "Add actions to perform in response to Process button being pressed"
        n173 = Decimal String To Number(string=w414) -> (number=w413:i32)  [unwired: 2 in, 1 out]
        n174 = Not Equal To 0?(x=w413) -> (x != 0?=w407:bool)
        n175 = call "PfeifferMVP15.vi"("On?"=w407, "Write?"=TRUE, "error in"=w406, "Cmd"=w403, "Adress"=u16 2, "VISA session"=w411) -> ("error out"=w401:errorcluster, "Result"=w405:variant, "VISA session Out"=w410:refnum<visa-resource-name>)  [unwired: 3 in]
        n176 = Insert Into Map(map in=w404, key=w403, value=w405) -> (map out=w402:map{T3, variant})  [unwired: 2 out]
      }
      frame "MnMVPStdBy" {
        w418 = PfeifferMVP15Cmds."Standby" ("Cmd")
        # "Add actions to perform in response to Process button being pressed"
        n177 = Decimal String To Number(string=w429) -> (number=w428:i32)  [unwired: 2 in, 1 out]
        n178 = Not Equal To 0?(x=w428) -> (x != 0?=w422:bool)
        n179 = call "PfeifferMVP15.vi"("On?"=w422, "Write?"=TRUE, "error in"=w421, "Cmd"=w418, "Adress"=u16 2, "VISA session"=w426) -> ("error out"=w416:errorcluster, "Result"=w420:variant, "VISA session Out"=w425:refnum<visa-resource-name>)  [unwired: 3 in]
        n180 = Insert Into Map(map in=w419, key=w418, value=w420) -> (map out=w417:map{T3, variant})  [unwired: 2 out]
      }
      frame "AckErrors" {
        w432 = TRUE ("Write?")
        w440 = PfeifferTC110Cmds."AckError" ("CMD ID")
        n181 = call "PfeifferTC110.vi"("Write?"=w432, "error in"=w444, "Adress"=u16 1, "VISA session"=w446, "CMD ID"=w440) -> ("error out"=w438:errorcluster, "VISA session out"=w441:refnum<visa-resource-name>)  [unwired: 4 in, 1 out]
        n182 = call "PfeifferTC110.vi"("Write?"=w432, "error in"=w438, "Adress"=u16 3, "VISA session"=w441, "CMD ID"=w440) -> ("error out"=w436:errorcluster, "VISA session out"=w437:refnum<visa-resource-name>)  [unwired: 4 in, 1 out]
        n183 = case shown="True" FALSE {
          tunnel: w437 -> [w448 w455]
          tunnel: w436 -> [w447 w452]
          tunnel: [w447 w451] -> w435
          tunnel: [w448 w450] -> w433
          tunnel: w432 -> [_ w449]
          frame False {
          }
          frame True {
            n184 = call "PfeifferMVP15.vi"("Write?"=w449, "error in"=w452, "Cmd"=PfeifferMVP15Cmds."AckError", "Adress"=u16 2, "VISA session"=w455) -> ("error out"=w451:errorcluster, "VISA session Out"=w450:refnum<visa-resource-name>)  [unwired: 4 in, 1 out]
          }
        }
      }
    }
  }
  n185 = call <userlib>:"MGI Exit if Runtime.vi"("Error In (Dependency Only)"=w10) -> ()  [unwired: 11 in]
